vi "Pre Launch Init.vi"(11 "Ex Nested in":refnum<class "Instrument Actor.lvclass">) -> (0 "error out":errorcluster, 3 "Ex Nested out":refnum<class "Instrument Actor.lvclass">)   [LabVIEW 2016, in "Instrument Actor.lvclass"]
doc: "(<B>Filename</B>: Actor Framework.lvlib:Actor.lvclass:Pre Launch Init.vi)\n\nDefines behavior that occurs after the Launch Nested Actor method is invoked but before the actor's Actor Core method begins running.\n\nBy default, this method does nothing. A descendant class may override it to define behavior."
uses:
  Instrument Actor.lvclass
  Command/Command.lvclass
  state.ctl
  Data/Data.lvclass
  Session APIs/File Access/Config Data/Config Data.lvclass
  G:/sw_repo/For Builds/Reusable/Session APIs/_Session Fwk/Session - Root.lvclass
  Session APIs/Session Log/System Log.lvclass
  cvt_update.ctl
  Session APIs/File Access/Config Data/Config Data.lvclass/Config Data.ctl
  Session APIs/Session Log/System Log.lvclass/System Log.ctl
  Instrument Actor.lvclass/Instrument Actor.ctl
  Instrument.lvclass/Instrument.ctl
  Write CMD.vi
  Write Log Session.vi
  Write Cfg Session.vi
  Write Data Notifier.vi
  Write ExtCom.vi
  Session APIs/Session Log/Accessors/Write Main Path.vi
  Session APIs/File Access/Config Data/Accessors/Write Cfg Path.vi
  SuperActor/xGlobal Data.vi
  SuperActor/SuperActor.lvclass
  Instrument.lvclass
  Session APIs/_Session Fwk/Session - Root.lvclass
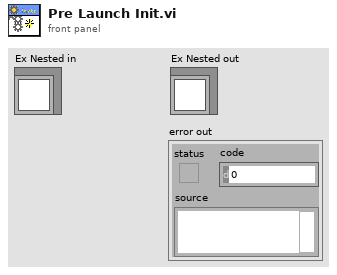
[diagram p1: front panel]
types:
  T1 = typedef "cvt_update.ctl" = cluster{"tag":string, "section":string, "value":variant}
  T2 = typedef "Instrument.lvclass/state.ctl" = enum8{"Configure", "Acquire", "Wait", "Quit", "Handle Error", "NOOP"}
  T3 = typedef "Session - Root.lvclass/Session Handle.ctl" = refnum<data-value>
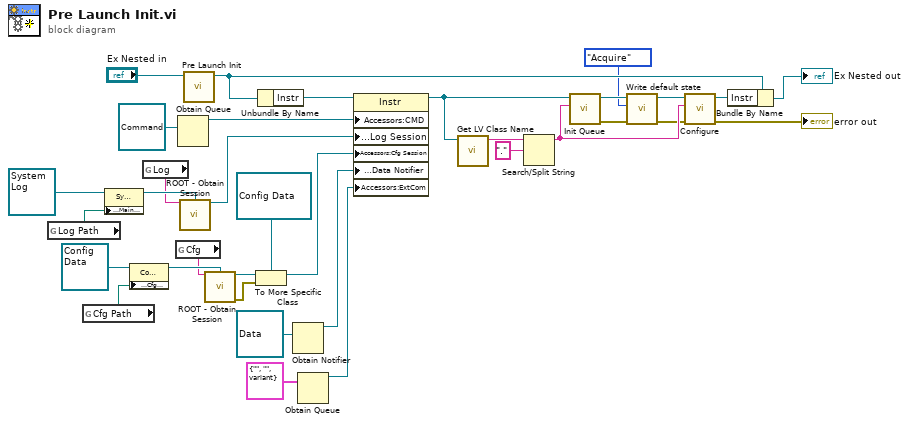
[diagram p0: block diagram]
diagram:
  n1 = global read "xGlobal Data.vi" "Log Path"() -> (w2:path)
  n2 = global read "xGlobal Data.vi" "Cfg Path"() -> (w1:path)
  n3 = property class="Sys Log"(reference=refnum<class "System Log.lvclass"> refnum ("Sys Log"), "Accessors:Main Path"=w2) -> (reference out=w15:refnum<class "System Log.lvclass">)  [unwired: 1 in, 1 out]
  n4 = property class="Config Data"(reference=refnum<class "Config Data.lvclass"> refnum ("Config Data"), "Accessors:Cfg Path"=w1) -> (reference out=w17:refnum<class "Config Data.lvclass">)  [unwired: 1 in, 1 out]
  n5 = global read "xGlobal Data.vi" "Log"() -> (w4:string)
  n6 = global read "xGlobal Data.vi" "Cfg"() -> (w3:string)
  n7 = Obtain Queue(element data type=refnum<class "Command.lvclass"> refnum ("CMD")) -> (queue out=w31:refnum<queue>)  [unwired: 4 in, 2 out]
  n8 = call "ROOT - Obtain Session.vi"("Session Name ()"=w4, "OBJ - Session"=w15) -> ("Session Handle"=w14:T3)  [unwired: 11 in, 2 out]
  n9 = call-parent "Pre Launch Init.vi"("Ex Nested in"="Ex Nested in") -> ("Ex Nested out"=w30:refnum<class "Instrument Actor.lvclass">)  [unwired: 9 in, 1 out]
  n10 = call "ROOT - Obtain Session.vi"("Session Name ()"=w3, "OBJ - Session"=w17) -> ("Session Handle"=w12:T3, "error out"=w13:errorcluster)  [unwired: 11 in, 1 out]
  n11 = To More Specific Class(target class=refnum<data-value> refnum, reference=w12, error in=w13) -> (specific class reference=w10:refnum<data-value>)  [unwired: 1 out]
  n12 = Unbundle By Name(w30) -> ("Instr"=w32:refnum<class "Instrument.lvclass">)
  n13 = Obtain Notifier(notification data type=refnum<class "Data.lvclass"> refnum ("Base Data Lib:Data")) -> (notifier out=w20:refnum<notifier>)  [unwired: 3 in, 2 out]
  n14 = Obtain Queue(element data type=T1 {"tag"="", "section"="", "value"=variant}) -> (queue out=w5:refnum<queue>)  [unwired: 4 in, 2 out]
  n15 = property class="Instr"(reference=w32, "Accessors:CMD"=w31, "Accessors:Log Session"=w14, "Accessors:Cfg Session"=w10, "Accessors:Data Notifier"=w20, "Accessors:ExtCom"=w5) -> (reference out=w26:refnum<class "Instrument.lvclass">)  [unwired: 1 in, 1 out]
  n16 = call <vilib>:"Get LV Class Name.vi"("object"=w26) -> ("class name"=w28:string)  [unwired: 9 in, 1 out]
  n17 = Search/Split String(string=w28, search string/char (-)="." ("regular expression")) -> (substring before match=w22:string)  [unwired: 1 in, 2 out]
  n18 = call "Init Queue.vi"("queue_name"=w22, "Instrument in"=w26) -> ("error out"=w8:errorcluster, "Instrument out"=w25:refnum<class "Instrument.lvclass">)  [unwired: 8 in]
  n19 = call "Write default state.vi"("error in (no error)"=w8, "instr state"=state."Acquire", "Instrument in"=w25) -> ("error out"=w7:errorcluster, "Instrument out"=w23:refnum<class "Instrument.lvclass">)  [unwired: 7 in]
  n20 = call-dynamic "Configure.vi"("error in"=w7, "name"=w22, "Instrument in"=w23) -> ("error out"=→"error out":errorcluster, "Instrument out"=w16:refnum<class "Instrument.lvclass">)  [unwired: 7 in]
  n21 = Bundle By Name(cluster=w30, "Instr"=w16) -> (→"Ex Nested out":refnum<class "Instrument Actor.lvclass">)
